vi "Actor Core.vi"(8 "error in":errorcluster, 11 "Dynamic Filter Window in":refnum<class "Dynamic Filter Window.lvclass">) -> (0 "error out":errorcluster, 3 "Actor out":refnum<class "Actor.lvclass">)   [LabVIEW 2018, in "Assert API Components.lvlib" / "Assert Display.lvlib" / "Main Display.lvlib" / "Dynamic Filter Window.lvlib" / "Dynamic Filter Window.lvclass"]
doc: "(<B>Filename</B>: Actor Framework.lvlib:Actor.lvclass:Actor Core.vi)\n\nReceives messages to the actor, reacts to them, and initiates any error handling that may shut the actor down.\n\nDescendant classes may override this VI to append parallel tasks for the actor to complete while it handles messages. Overrides use the Call Parent Method node."
uses:
  Dynamic Filter Window.lvclass
  C:/Program Files (x86)/National Instruments/LabVIEW 2018/vi.lib/ActorFramework/Actor/Actor.lvclass
  C:/Users/UKHornP/Documents/Work/Projects/Assert API/Core/Base UI Actor/Base UI Actor/Base UI Actor.lvclass
  <vilib>/ActorFramework/Actor/Actor.lvclass
  Core/Assert API Components/Filter By String.ctl
  Core/Assert API Components/Filter Type.ctl
  Core/Assert API Components/Filter By Time.ctl
  <vilib>/ActorFramework/Actor/Actor.lvclass/Actor.ctl
  Core/Base UI Actor/Base UI Actor/Base UI Actor.lvclass/Base UI Actor.ctl
  <vilib>/ActorFramework/Message Enqueuer/Message Enqueuer.lvclass/Message Enqueuer.ctl
  Core/Assert API Components/Boolean Filter Configuration.ctl
  Core/Assert API Components/Time Filter Configuration.ctl
  Core/Assert API Components/String Filter Configuration.ctl
  Core/Assert API Components/Filter Configurations/Base Filter.lvclass/Base Filter.ctl
  Core/Main Display/Main Display Messages/Configure Filter Msg/Configure Filter Msg.lvclass/Configure Filter Msg.ctl
  Core/Main Display/Main Display Messages/Remove Named Filter Msg/Remove Named Filter Msg.lvclass/Remove Named Filter Msg.ctl
  <vilib>/ActorFramework/Message Enqueuer/Init from Existing Queue.vi
  <vilib>/ActorFramework/Message Enqueuer/Enqueue.vi
  Core/Main Display/Main Display Messages/Configure Filter Msg/Configure Filter Msg.lvclass
  C:/Program Files (x86)/National Instruments/LabVIEW 2018/vi.lib/ActorFramework/Message/Message.lvclass
  Core/Main Display/Main Display Messages/Remove Named Filter Msg/Remove Named Filter Msg.lvclass
  <vilib>/ActorFramework/Stop Msg/Stop Msg.lvclass
  <vilib>/Utility/LVClass/Get LV Class Name.vi
  <resource>/AFDebug/Generate Trace for Message.vi
  <vilib>/ActorFramework/Message Priority Queue/Priority Enqueue.vi
  Core/Base UI Actor/Base UI Actor/Base UI Actor.lvclass
  <vilib>/ActorFramework/Message Enqueuer/Message Enqueuer.lvclass
  Core/Assert API Components/Filter Configurations/Base Filter.lvclass
  Core/Assert Display/Assert Display.lvlib
panel:
  in  "Remove Filter Button":bool
  in  "Status":bool
  in  "Time Comparison Method":enum16{"Before", "After"}(ring)
  in  "Update Filter Button":bool
  in  "Time Stamp":timestamp
  in  "Filter Time":T1
  in  "Filter Type":T2
  in  "Filter String":T3
  in  "Include or Exclude":enum16{"Include", "Exclude"}(ring)
  in  "String Comparison Method":T4(ring)
  in  "Comparison Value":string
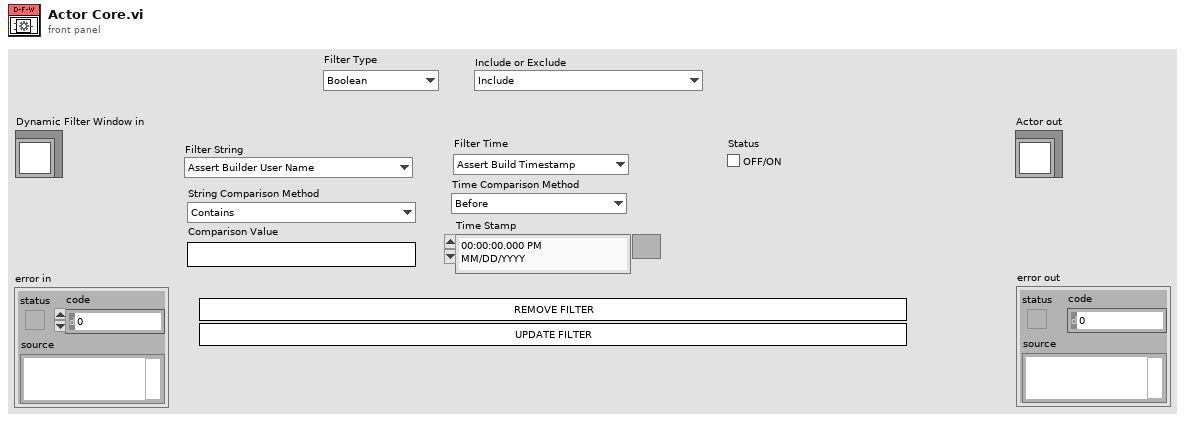
[diagram p1: front panel]
types:
  T1 = typedef "Assert API Components.lvlib/Assert Display.lvlib/Filter By Time.ctl" = enum16{"Assert Build Timestamp", "Last Update Timestamp"}
  T2 = typedef "Assert API Components.lvlib/Assert Display.lvlib/Filter Type.ctl" = enum16{"Boolean", "String", "Time"}
  T3 = typedef "Assert API Components.lvlib/Assert Display.lvlib/Filter By String.ctl" = enum16{"Assert Builder User Name", "Assert Name", "Assert VI Name", "Calling VI Name", "Comment", "Data Type", "Evaluation String"}
  T4 = enum16{"Contains", "Does Not Contain", "Starts With", "Equals", "Does Not Equal"}
  T5 = typedef "Assert API Components.lvlib/Assert Display.lvlib/String Filter Configuration.ctl" = cluster{"Filter String":T3, "String Comparison Method":enum16{"Contains", "Does Not Contain", "Starts With", "Equals", "Does Not Equal"}, "Comparison Value":string}
  T6 = typedef "Assert API Components.lvlib/Assert Display.lvlib/Time Filter Configuration.ctl" = cluster{"Filter Time":T1, "Time Comparison Method":enum16{"Before", "After"}, "Time Stamp":timestamp}
  T7 = typedef "Assert API Components.lvlib/Assert Display.lvlib/Boolean Filter Configuration.ctl" = cluster{"Boolean Comparison Value":bool}
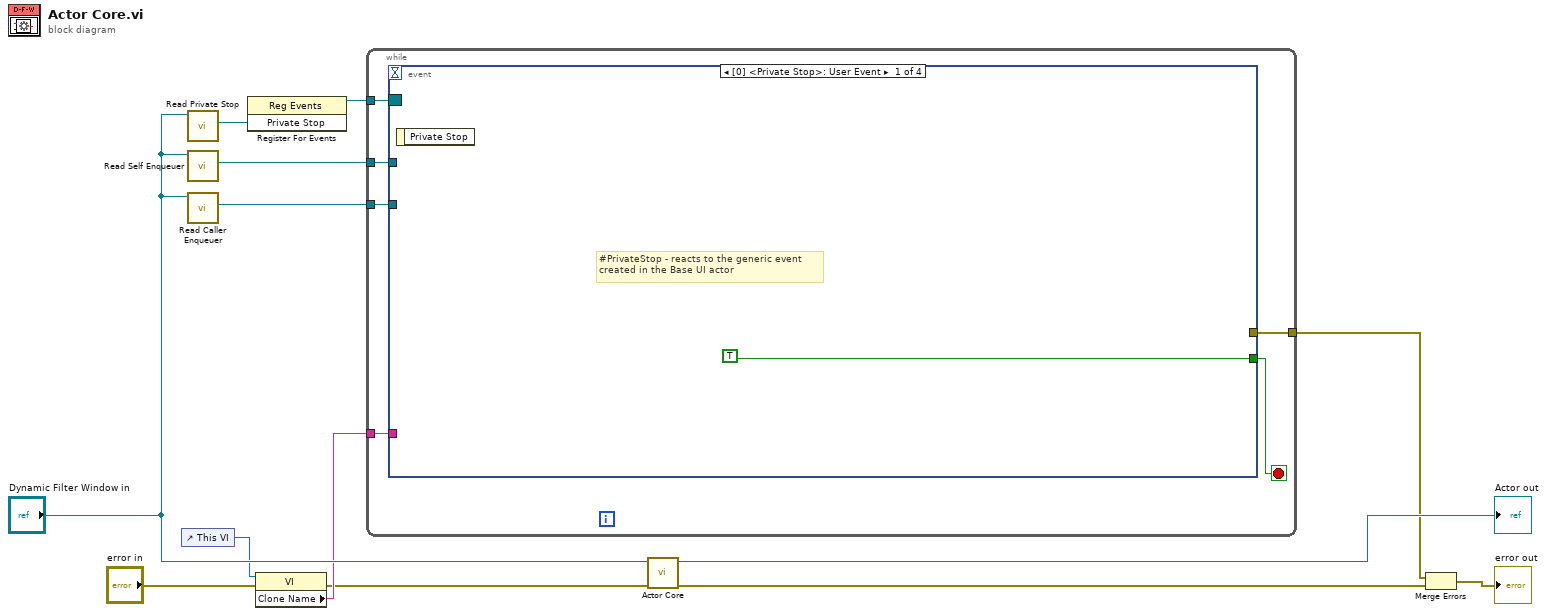
[diagram p0: block diagram]
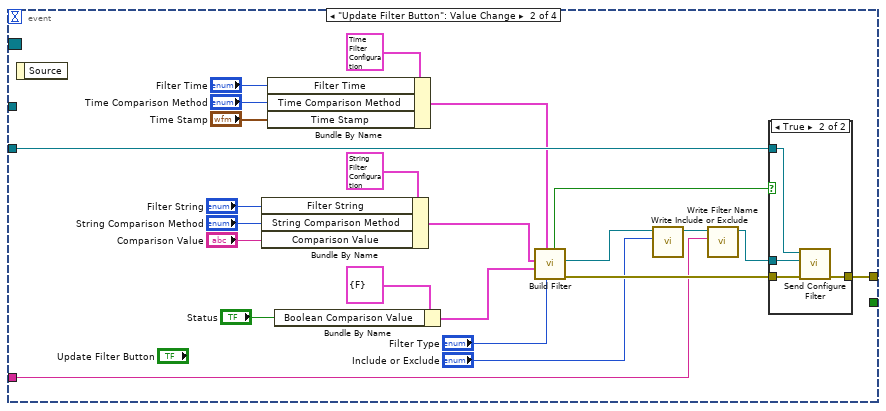
[diagram p2: hidden frame]
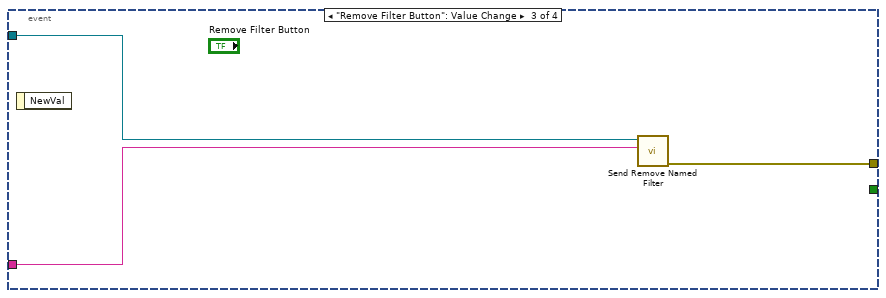
[diagram p4: hidden frame]
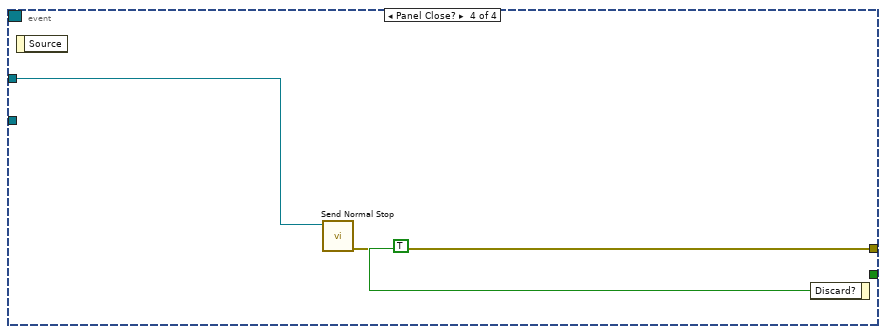
[diagram p5: hidden frame]
diagram:
  n1 = control-ref of="This VI"() -> (w6:refnum<vi>)
  n2 = call "Read Private Stop.vi"("Base UI Actor in"="Dynamic Filter Window in") -> ("Private Stop"=w11:refnum<user-event>)  [unwired: 10 in]
  n3 = call <vilib>:"Read Self Enqueuer.vi"("Actor"="Dynamic Filter Window in") -> ("Self Enqueuer"=w7:refnum<class "Message Enqueuer.lvclass">)  [unwired: 10 in]
  n4 = call <vilib>:"Read Caller Enqueuer.vi"("Actor"="Dynamic Filter Window in") -> ("Caller Enqueuer"=w9:refnum<class "Message Enqueuer.lvclass">)  [unwired: 10 in]
  n5 = register-events(w11) -> (reference out=w10:refnum<event-registration>)  [unwired: 2 in, 1 out]
  n6 = property class="VI"(reference=w6, error in="error in") -> (error out=w3:errorcluster, "Clone Name"=w5:string)  [unwired: 1 out]
  n7 = while {
    tunnel: w10 -> [w19]
    tunnel: w9 -> [w17]
    tunnel: w7 -> [w16]
    tunnel: w5 -> [w15]
    tunnel: [w14] -> w1
    stop <- w18 stop-if-true
    n8 = event shown="[0] <Private Stop>: User Event" {
      selector: w19 -> [_ _ _ _]
      dyn-events: _ -> [_ _ _ _]
      timeout: _ -> [_ _ _ _]
      tunnel: [TRUE _ _ _] -> w18
      tunnel: w17 -> [_ w42 w51 _]
      tunnel: w16 -> [_ _ _ w53]
      tunnel: w15 -> [_ w37 w50 _]
      tunnel: [_ w41 w49 w52] -> w14
      event User Event {
        # "#PrivateStop - reacts to the generic event created in the Base UI actor"
        n9 = event-data() -> ()  [unwired: 1 in, 1 out]
      }
      event "Update Filter Button": Value Change {
        n10 = event-data() -> ()  [unwired: 1 in, 1 out]
        n11 = Bundle By Name(cluster=T5 {"Filter String"=enum."Assert Builder User Name", "String Comparison Method"=enum."Contains", "Comparison Value"=""}, "Filter String"="Filter String", "String Comparison Method"="String Comparison Method", "Comparison Value"="Comparison Value") -> (w25:T5)
        n12 = Bundle By Name(cluster=T6 {"Filter Time"=enum."Assert Build Timestamp", "Time Comparison Method"=enum."Before", "Time Stamp"=timestamp(0 s since 1904-01-01)}, "Filter Time"="Filter Time", "Time Comparison Method"="Time Comparison Method", "Time Stamp"="Time Stamp") -> (w23:T6)
        n13 = Bundle By Name(cluster=T7 {"Boolean Comparison Value"=FALSE}, "Boolean Comparison Value"="Status") -> (w24:T7)
        n14 = call "Build Filter.vi"("Filter Type"="Filter Type", "Time Filter Configuration"=w23, "Boolean Filter Configuration"=w24, "String Filter Configuration"=w25) -> ("error out"=w43:errorcluster, "Base Filter out"=w30:refnum<class "Base Filter.lvclass">, "Boolean"=w22:bool)  [unwired: 5 in]
        n15 = call "Write Include or Exclude.vi"("Include or Exclude"="Include or Exclude", "Base Filter in"=w30) -> ("Base Filter out"=w39:refnum<class "Base Filter.lvclass">)  [unwired: 9 in]
        n16 = call "Write Filter Name.vi"("Filter Name"=w37, "Base Filter in"=w39) -> ("Base Filter out"=w38:refnum<class "Base Filter.lvclass">)  [unwired: 9 in]
        n17 = case shown="True" w22 {
          tunnel: w42 -> [_ w48]
          tunnel: [w44 w47] -> w41
          tunnel: w38 -> [_ w46]
          tunnel: w43 -> [w44 w45]
          frame False {
          }
          frame True {
            n18 = call "Send Configure Filter.vi"("error in (no error)"=w45, "New Filter"=w46, "Message Enqueuer"=w48) -> ("error out"=w47:errorcluster)  [unwired: 7 in, 1 out]
          }
        }
      }
      event "Remove Filter Button": Value Change {
        n19 = event-data() -> ()  [unwired: 1 in, 1 out]
        n20 = call "Send Remove Named Filter.vi"("Filter Name"=w50, "Message Enqueuer"=w51) -> ("error out"=w49:errorcluster)  [unwired: 8 in, 1 out]
      }
      event Panel Close? {
        n21 = event-data() -> ()  [unwired: 1 in, 1 out]
        n22 = call <vilib>:"Send Normal Stop.vi"("Message Enqueuer"=w53) -> ("error out"=w52:errorcluster)  [unwired: 10 in]
        n23 = event-data("Discard?"=TRUE) -> ()  [unwired: 1 in, 1 out]
      }
    }
  }
  n24 = call-parent "Actor Core.vi"("error in"=w3, "Actor in"="Dynamic Filter Window in") -> ("error out"=w13:errorcluster, "Actor out"=→"Actor out":refnum<class "Actor.lvclass">)  [unwired: 8 in]
  n25 = Merge Errors(w1, w13) -> (→"error out":errorcluster)
